vi "K to C (1D dbl).vi"(1 "K":dbl[](array[numeric])) -> (0 "C":dbl[](array[numeric]))   [LabVIEW 2012, in "Temp Converter.lvlib"]
doc: "VI名称：K to C。\n\n<B>输入端子K</B>: 输入开氏温度。\n<B>输出端子C</B>: 输出摄氏温度。\n\n公式： C=K-273.15.\n创建者：CSXCS_366"
uses:
  Temp Converter.lvlib
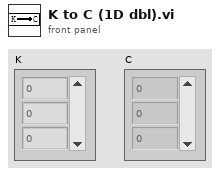
[diagram p1: front panel]
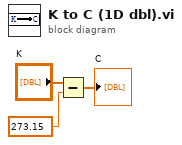
[diagram p0: block diagram]
diagram:
  n1 = Subtract(x="K", y=273.15) -> (x-y=→"C":dbl[])
